vi "Parse Request String.vi"(8 "error in (no error)":errorcluster, 9 "Request String":string) -> (0 "error out":errorcluster, 2 "Target URI":refnum<class "URI.lvclass">, 3 "Request out":refnum<class "Request.lvclass">)   [LabVIEW 2020, in "HTTP Utils.lvlib" / "Request.lvclass"]
uses:
  Request.lvclass
  <vilib>/IlluminatedG/lv-stream/URI/URI.lvclass
  Request.lvclass/Request.ctl
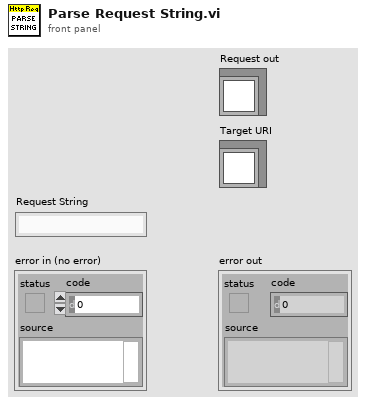
[diagram p1: front panel]
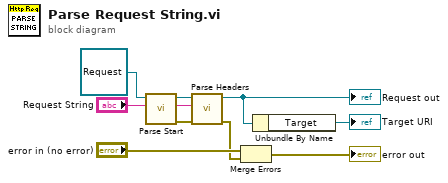
[diagram p0: block diagram]
diagram:
  n1 = call "Parse Start.vi"("String in"="Request String", "Request in"=refnum<class "Request.lvclass"> refnum) -> ("error out"=w5:errorcluster, "Remaining"=w6:string, "Request out"=w7:refnum<class "Request.lvclass">)  [unwired: 7 in]
  n2 = call "Parse Headers.vi"("error in (no error)"=w5, "String in"=w6, "Request in"=w7) -> ("error out"=w2:errorcluster, "Request out"=w1:refnum<class "Request.lvclass">)  [unwired: 7 in]
  "Request out" <- w1
  n3 = Merge Errors("error in (no error)", w2) -> (→"error out":errorcluster)
  n4 = Unbundle By Name(w1) -> ("Target"=→"Target URI":refnum<class "URI.lvclass">)
